vi "5.1 Act.vi"() -> ()   [LabVIEW 2010]
uses:
  4-High Neurons/4.0-Timing Badass.ctl
  4-High Neurons/4.1-Act Control Typedef.ctl
  6-OCU Neurons/6.1-UDP Saitek.ctl
  5.0-Global.vi
panel:
  out "length":i32
  out "type string":i16[](array[numeric])
  out "data string":string
  in  "stop":bool
  out "Super Heart Beat":T1
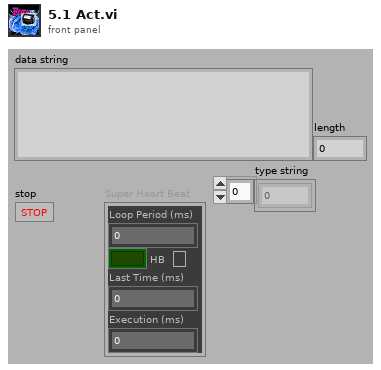
[diagram p1: front panel]
types:
  T1 = typedef "4.0-Timing Badass.ctl" = cluster{"Loop Period (ms)":u32, "HB":bool, "Last Time (ms)":u32, "Execution (ms)":u32}
  T2 = typedef "4.1-Act Control Typedef.ctl" = cluster{"E-Stop":bool, "Restart":bool, "Extended Joystick":bool, "Begin":bool, "Time":i32, "Shutdown":bool, "Saitek Controler":T3, "Joystick Valid":bool}
  T3 = typedef "6.1-UDP Saitek.ctl" = cluster{"Stop":bool, "Setpoint":bool, "Run":bool, "Restart":bool, "Shutdown":bool, "Joystick\nMode 1":bool, "Joystick\nMode 2":bool, "Joystick \nMode 3":bool, "Joystick Mode 4":bool, "10":bool, "11":bool, "Pitch":sgl, "Roll":sgl, "Yaw":sgl, "Left":sgl, "Right":sgl}
  T4 = typedef "6.1-Act.ctl" = cluster{"6.1-Saitek Controller":T3, "Joystick Mode":bool, "Shutdown":bool, "Reset":bool, "Begin":bool}
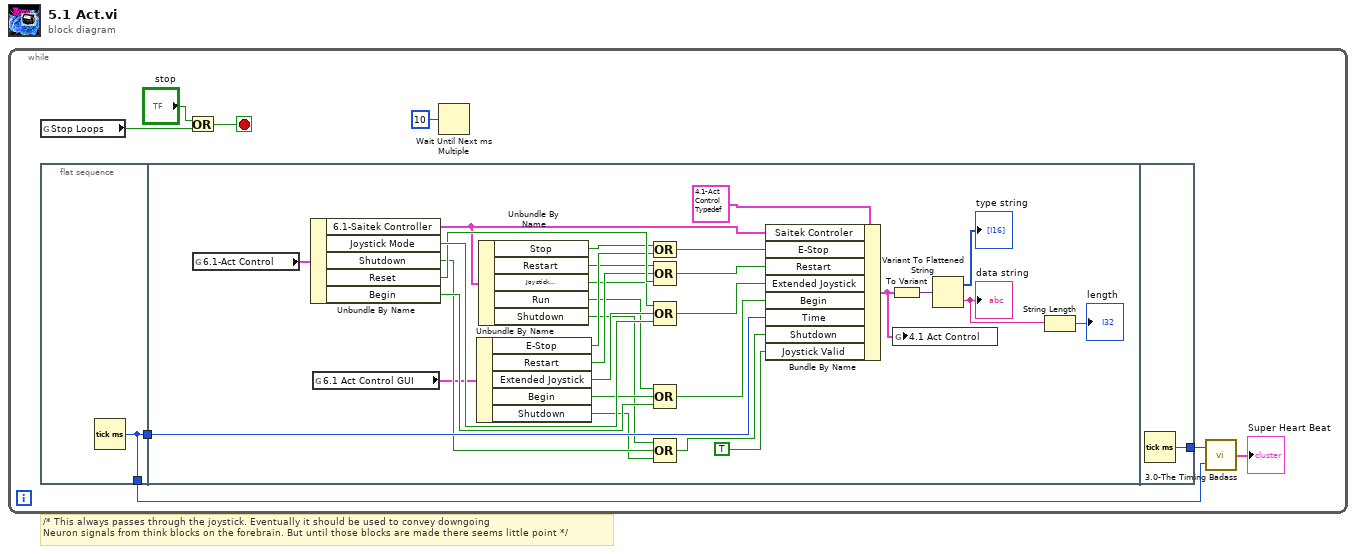
[diagram p0: block diagram]
diagram:
  # "/* This always passes through the joystick. Eventually it should be used to convey downgoing\nNeuron signals from think blocks on the forebrain. But until those blocks are made there seems little point */"
  n1 = while {
    stop <- w4 stop-if-true
    n2 = global read "5.0-Global.vi" "Stop Loops"() -> (w3:bool)
    n3 = flat-sequence {
      tunnel: [w9] -> w7
      tunnel: [w9] -> w2
      tunnel: w2 -> [w29]
      tunnel: [w40] -> w8
      frame #0 {
        n4 = Tick Count (ms)() -> (millisecond timer value=w9:u32)
      }
      frame #1 {
        n5 = global read "5.0-Global.vi" "6.1-Act Control"() -> (w38:T4)
        n6 = Unbundle By Name(w38) -> ("6.1-Saitek Controller"=w11:T3, "Joystick Mode"=w37:bool, "Shutdown"=w27:bool, "Reset"=w36:bool, "Begin"=w28:bool)
        n7 = global read "5.0-Global.vi" "6.1 Act Control GUI"() -> (w26:T2)
        n8 = Unbundle By Name(w26) -> ("E-Stop"=w20:bool, "Restart"=w19:bool, "Extended Joystick"=w18:bool, "Begin"=w17:bool, "Shutdown"=w16:bool)
        n9 = Unbundle By Name(w11) -> ("Stop"=w30:bool, "Restart"=w15:bool, "Joystick \nMode 3"=w14:bool, "Run"=w13:bool, "Shutdown"=w12:bool)
        n10 = Compound Arithmetic op=OR(w30, w20) -> (w25:bool)
        n11 = Compound Arithmetic op=OR(w15, w19, w36) -> (w24:bool)
        n12 = Compound Arithmetic op=OR(w14, w18, w37) -> (w23:bool)
        n13 = Compound Arithmetic op=OR(w13, w17, w28) -> (w22:bool)
        n14 = Compound Arithmetic op=OR(w12, w27, w16) -> (w21:bool)
        n15 = Bundle By Name(cluster=T2 {"E-Stop"=FALSE, "Restart"=FALSE, "Extended Joystick"=FALSE, "Begin"=FALSE, "Time"=0, "Shutdown"=FALSE, "Saitek Controler"={"Stop"=FALSE, "Setpoint"=FALSE, "Run"=FALSE, "Restart"=FALSE, "Shutdown"=FALSE, "Joystick\nMode 1"=FALSE, "Joystick\nMode 2"=FALSE, "Joystick \nMode 3"=FALSE, "Joystick Mode 4"=FALSE, "10"=FALSE, "11"=FALSE, "Pitch"=0.0, "Roll"=0.0, "Yaw"=0.0, "Left"=0.0, "Right"=0.0}, "Joystick Valid"=FALSE} ("4.1 Act Control"), "Saitek Controler"=w11, "E-Stop"=w25, "Restart"=w24, "Extended Joystick"=w23, "Begin"=w22, "Time"=w29, "Shutdown"=w21, "Joystick Valid"=TRUE) -> (w35:T2)
        n16 = To Variant(anything=w35) -> (Variant=w34:variant)
        n17 = global write "5.0-Global.vi" "4.1 Act Control"(w35) -> ()
        n18 = Variant To Flattened String(Variant=w34) -> (data string=w32:string, 1:→"type string":i16[])
        "data string" <- w32
        n19 = String Length(string=w32) -> (length=→"length":i32)
      }
      frame #2 {
        n20 = Tick Count (ms)() -> (millisecond timer value=w40:u32)
      }
    }
    n21 = Or(x="stop", y=w3) -> (x .or. y?=w4:bool)
    n22 = Wait Until Next ms Multiple(millisecond multiple=u32 10) -> ()  [unwired: 1 out]
    n23 = call "3.0-The Timing Badass.vi"("Start"=w7, "End"=w8) -> ("Super Heart Beat"=→"Super Heart Beat":T1)
  }
